vi "DELETE Deviation Signal Data.vi"   [LabVIEW 2013]
uses:
  Functional Globals/Action.ctl
types:
  T1 = typedef "Action.ctl" = enum16{"GET", "PUT", "DELETE"}
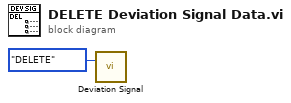
[diagram p0: block diagram]
diagram:
  n1 = call "Deviation Signal.vi"("Action"=Action."DELETE") -> ()  [unwired: 2 in, 1 out]
